vi "Set All Joint Positions.vi"(8 "error in (no error)":errorcluster, 9 "Body Index":i32, 10 "Joints":refnum<k24>, 11 "KinectSensor Reference":refnum<k24>) -> (0 "error out":errorcluster)   [LabVIEW 2011, in "KinectOne.lvlib"]
uses:
  KinectOne.lvlib
  Microsoft.Kinect
  Type Defs/JointType.ctl
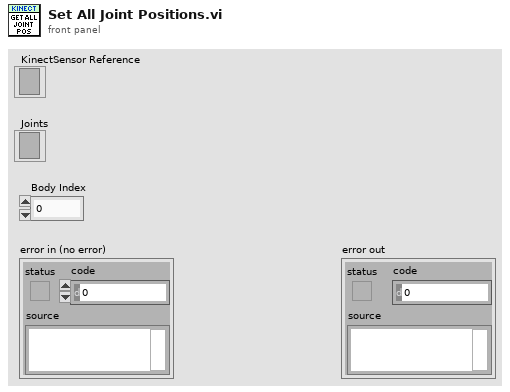
[diagram p1: front panel]
types:
  T1 = enum16{"Get Joint Position", "Initialize", "Set Joint Position"}
  T2 = typedef "KinectOne.lvlib/JointType.ctl" = i32
  T3 = typedef "KinectOne.lvlib/Joint Position.ctl" = cluster{"Color Space Position":cluster{"X":sgl, "Y":sgl}, "Depth Space Position":cluster{"X":sgl, "Y":sgl}, "TrackingState":i32}
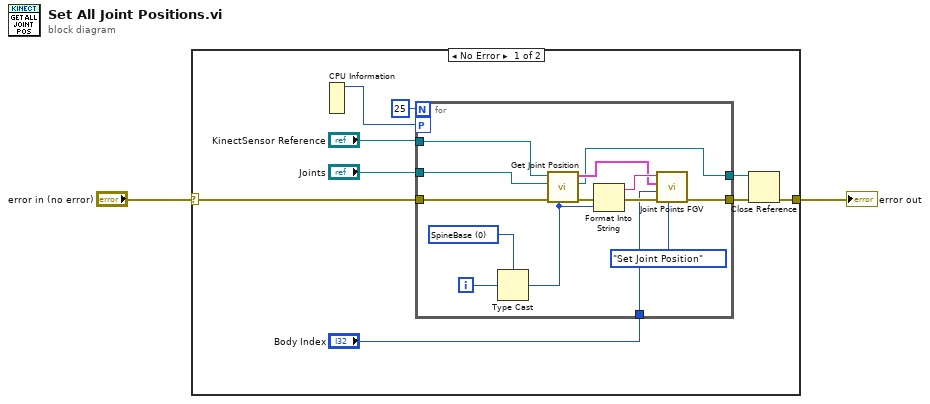
[diagram p0: block diagram]
diagram:
  n1 = case shown="No Error" "error in (no error)" {
    selector: "error in (no error)" -> [w6 w26]
    tunnel: [w5 w26] -> w2
    frame No Error {
      n2 = CPU Information() -> (4:w7:i32)  [unwired: 3 out]
      n3 = for {
        N: 25 -> [_]
        tunnel: "KinectSensor Reference" -> [w22]
        tunnel: "Joints" -> [w23]
        tunnel: w6 -> [w24]
        tunnel: [w17] -> w4
        workers-P: w7 -> [_]
        tunnel: "Body Index" -> [w15]
        tunnel: [w13] -> w3
        i -> [w25]
        w12 = T2 0 items=["SpineBase", "SpineMid", "Neck", "Head", "ShoulderLeft", "ElbowLeft", "WristLeft", "HandLeft", "ShoulderRight", "ElbowRight", "WristRight", "HandRight", "HipLeft", "KneeLeft", "AnkleLeft", "FootLeft", "HipRight", "KneeRight", "AnkleRight", "FootRight", "SpineShoulder", "HandTipLeft", "ThumbLeft", "HandTipRight", "ThumbRight"] ("JointType")
        n4 = Type Cast(type=w12, x=w25) -> (*(type *) &x=w14:T2)
        n5 = call "Get Joint Position.vi"("JointType"=w14, "error in (no error)"=w24, "Joints"=w23, "KinectSensor Reference"=w22) -> ("error out"=w19:errorcluster, "3856ad364e35]], mscorlib, Version=0.0.0.0, Culture=neutral, PublicKeyToken=b77a5c561934e089\nJoints out"=w13:refnum<k24>, "Joint Position"=w18:T3)  [unwired: 5 in]
        n6 = Format Into String(error in=w19, w14) -> (resulting string=w21:string, error out=w20:errorcluster)  [unwired: 2 in]
        n7 = call "Joint Points FGV.vi"("Command"=T1."Set Joint Position", "error in (no error)"=w20, "Body Index"=w15, "Joint Position"=w18, "name"=w21) -> ("error out"=w17:errorcluster)  [unwired: 5 in, 1 out]
      }
      n8 = Close Reference(reference=w3, error in (no error)=w4) -> (error out=w5:errorcluster)
    }
    frame Error {
    }
  }
  "error out" <- w2
